vi "Get Server DLL Path.vi"() -> (0 "Server dll path":path)   [LabVIEW 2019, in "gprc-lvsupport.lvlib"]
uses:
  gprc-lvsupport.lvlib
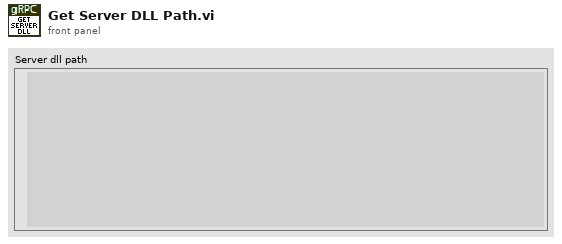
[diagram p1: front panel]
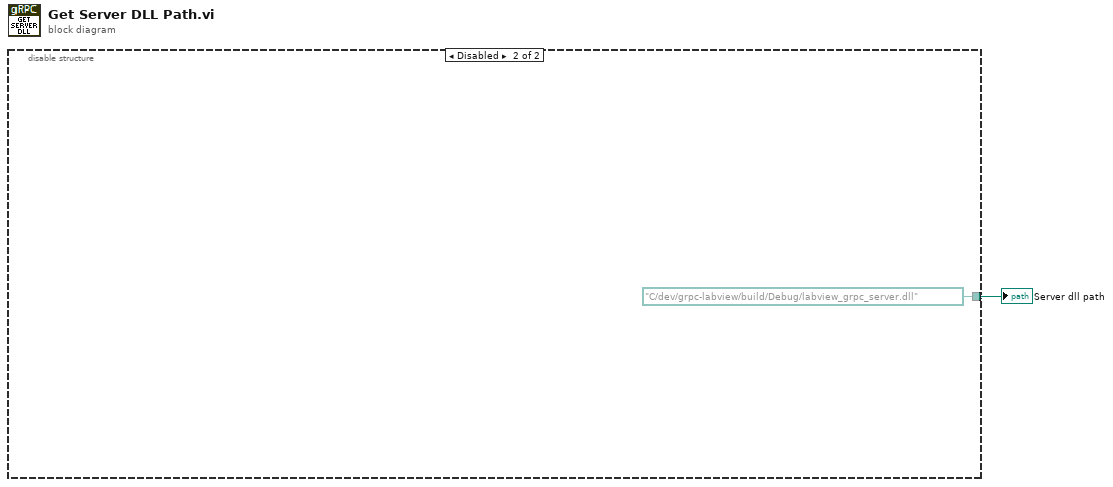
[diagram p0: block diagram]
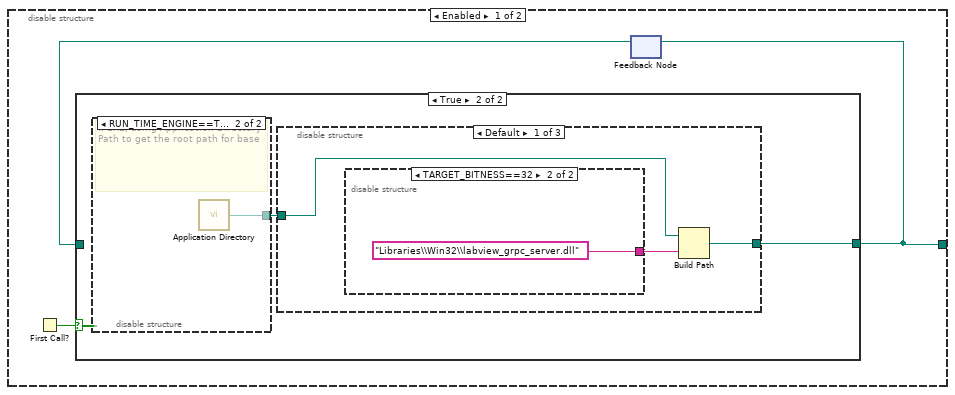
[diagram p2: hidden frame]
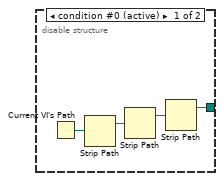
[diagram p4: hidden frame]
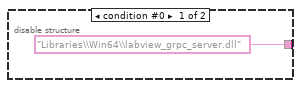
[diagram p5: hidden frame]
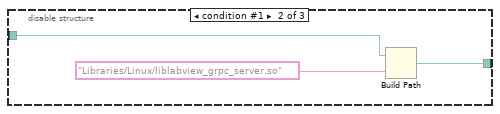
[diagram p6: hidden frame]
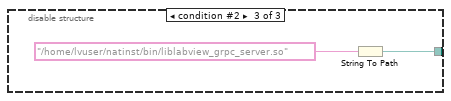
[diagram p7: hidden frame]
diagram:
  n1 = disable-structure shown="Disabled" {
    disable-tunnel: [w3 path "C:/dev/grpc-labview/build/Debug/labview_grpc_server.dll" ("Server dll path")] -> w1
    frame Enabled {
      n2 = First Call?() -> (First Call?: T/F=w4:bool)
      n3 = feedback #1() -> (w2:path)  [unwired: 1 in]
      n4 = case shown="True" w4 {
        tunnel: [w5 w6] -> w3
        tunnel: w2 -> [w5 _]
        frame False {
        }
        frame True {
          n5 = disable-structure shown="RUN_TIME_ENGINE==True" {
            disable-tunnel: [w8 w12] -> w7
            frame condition #0 (active) {
              n6 = Current VI's Path() -> (path=w10:path)
              n7 = Strip Path(path=w10) -> (stripped path=w11:path)  [unwired: 1 out]
              n8 = Strip Path(path=w11) -> (stripped path=w9:path)  [unwired: 1 out]
              n9 = Strip Path(path=w9) -> (stripped path=w8:path)  [unwired: 1 out]
            }
            frame condition #1 {
              # "If EXE, using Application Directory Path to get the root path for base"
              n10 = call <vilib>:"Application Directory.vi"() -> ("Application Directory"=w12:path)
            }
          }
          n11 = disable-structure shown="Default" {
            disable-tunnel: w7 -> [w14 w20 _]
            disable-tunnel: [w13 w19 w21] -> w6
            frame condition #0 (active) {
              n12 = disable-structure shown="TARGET_BITNESS==32" {
                disable-tunnel: ["Libraries\\Win64\\labview_grpc_server.dll" ("name or relative path") "Libraries\\Win32\\labview_grpc_server.dll" ("name or relative path")] -> w15
                frame condition #0 {
                }
                frame condition #1 (active) {
                }
              }
              n13 = Build Path(base path=w14, name or relative path=w15) -> (appended path=w13:path)
            }
            frame condition #1 {
              n14 = Build Path(base path=w20, name or relative path="Libraries/Linux/liblabview_grpc_server.so") -> (appended path=w19:path)
            }
            frame condition #2 {
              n15 = String To Path(string="/home/lvuser/natinst/bin/liblabview_grpc_server.so" ("name or relative path")) -> (path=w21:path)
            }
          }
        }
      }
      n16 = feedback-in #1(w3) -> ()
    }
    frame Disabled {
    }
  }
  "Server dll path" <- w1
